vi "FF_compute2_Moiz.vi"(1 "GaitCylce(%)":dbl, 4 "Boolean":bool, 6 "FrameNum":dbl, 8 "xyz_o":dbl[][](array[numeric]), 10 "CenPt":dbl[](array[numeric]), 11 "Array":T1[](array[typedef])) -> (0 "Closest Pt":dbl[](array[numeric]), 2 "DesiredFM_FF":dbl[](array[numeric]), 3 "ForceAll":dbl[][](array[numeric]), 5 "curr Point":dbl[](array[numeric]), 9 "TraFF":dbl[](array[numeric]))   [LabVIEW 2013]
uses:
  typeDef/AnkleTraj.ctl
  <vilib>/Analysis/baseanly.llb/Real Dot Product.vi
  <vilib>/Analysis/_algsub.llb/Real Vector Norm.vi
  <vilib>/Analysis/BLAS.llb/idamin - Min Element Index (DBL).vi
  <vilib>/Analysis/NI_AALBase.lvlib
  <vilib>/Analysis/NI_AALPro.lvlib
  <vilib>/Analysis/NI_AALBLAS.lvlib
panel:
  out "Out of first loop":T1[](array[typedef])
  in  "FF Constant":T2
  in  "HalfWindow FF 2":i32=60
  out "x < y?":bool
  out "Array 2":i32[](array[numeric])
  out "P1FF":dbl[](array[numeric])
  out "P1 full size":i32[](array[numeric])
  out "P2 full":dbl[][](array[numeric])
  out "P1 full":dbl[][](array[numeric])
  out "CheckPlus":dbl[][](array[numeric])
  in  "AnkleTraj":T1
  out "HalfWindow FF":i32
  out "P'":dbl[](array[numeric])
  out "Array 4":dbl[](array[numeric])
  out "OrderOfClosePt":i32
  in  "DesiredM_FF":dbl[](array[numeric])=[5.0, 5.0, 5.0, 4.0, 4.0, 4.0]
  in  "Enum":enum16{"Linear", "Bell"}(ring)=enum."Bell"
  out "ForceComp":dbl[](array[numeric])
  out "n_dir":dbl[](array[numeric])
  out "d_min":dbl
  out "ForceXYZ":dbl[](array[numeric])
  out "TangentVectorAtClosestPt":dbl[](array[numeric])
  out "NormalVectorToClosestPt":dbl[](array[numeric])
  out "DistanceToClosestPt":dbl
  out "IndexOfClosePt":i32
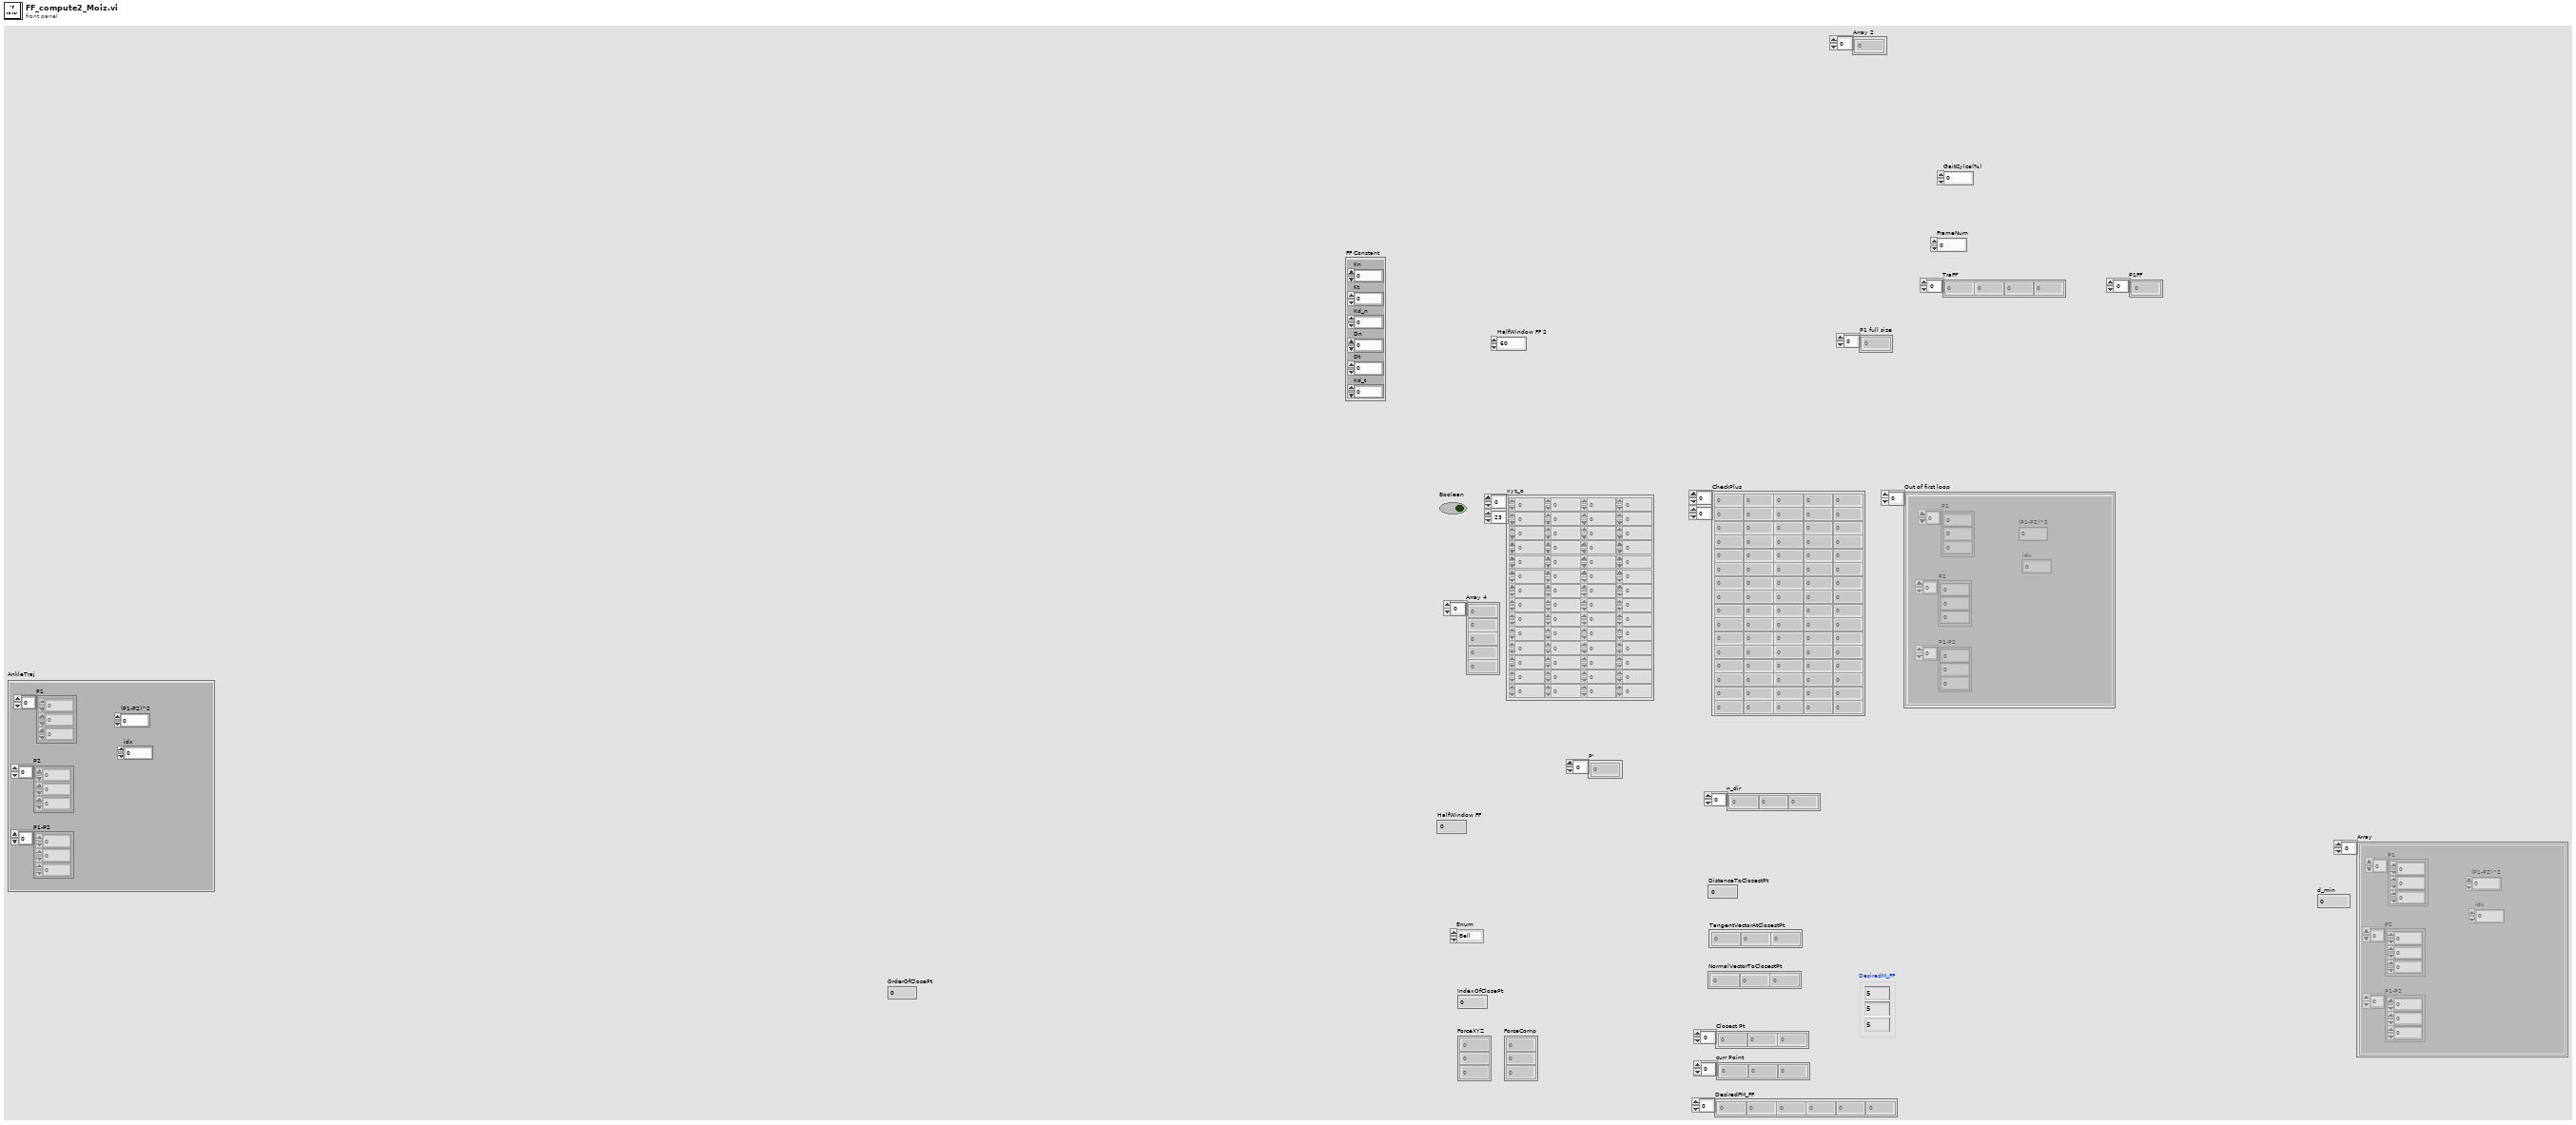
[diagram p1: front panel]
types:
  T1 = typedef "AnkleTraj.ctl" = cluster{"P1":dbl[], "P2":dbl[], "P1-P2":dbl[], "(P1-P2)^2":dbl, "idx":i32}
  T2 = cluster{"Kn":dbl, "Kt":dbl, "Kd_n":dbl, "Dn":dbl, "Dt":dbl, "Kd_t":dbl}
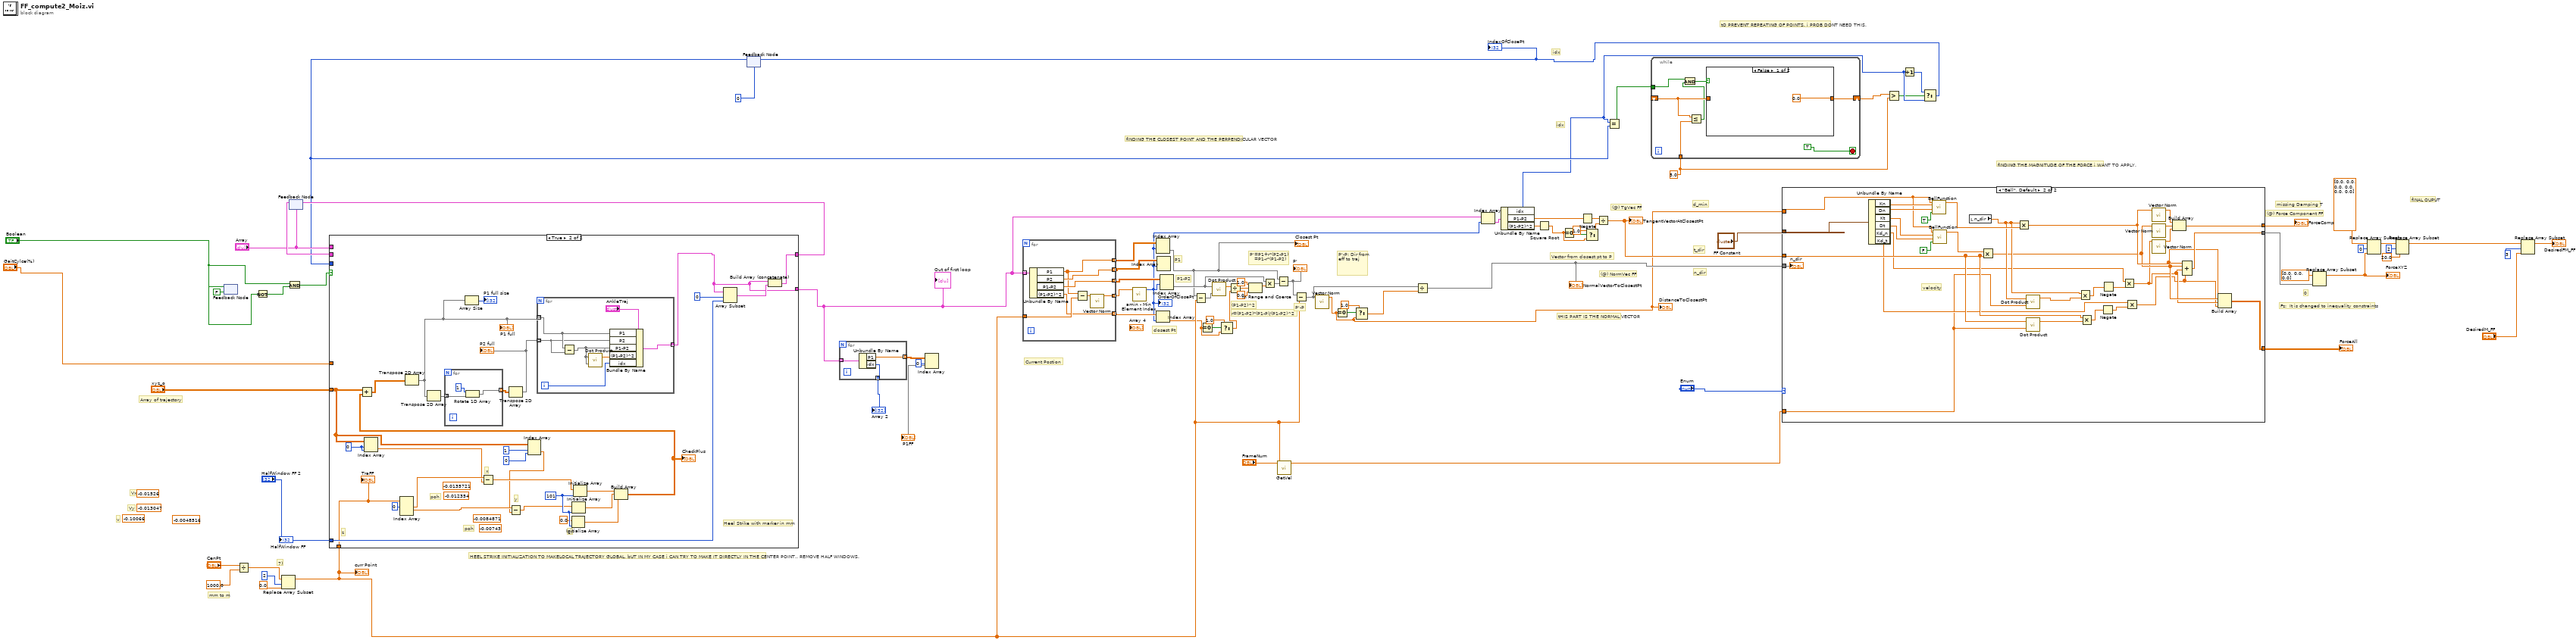
[diagram p0: block diagram]
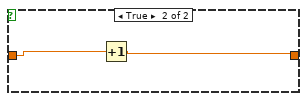
[diagram p2: hidden frame]
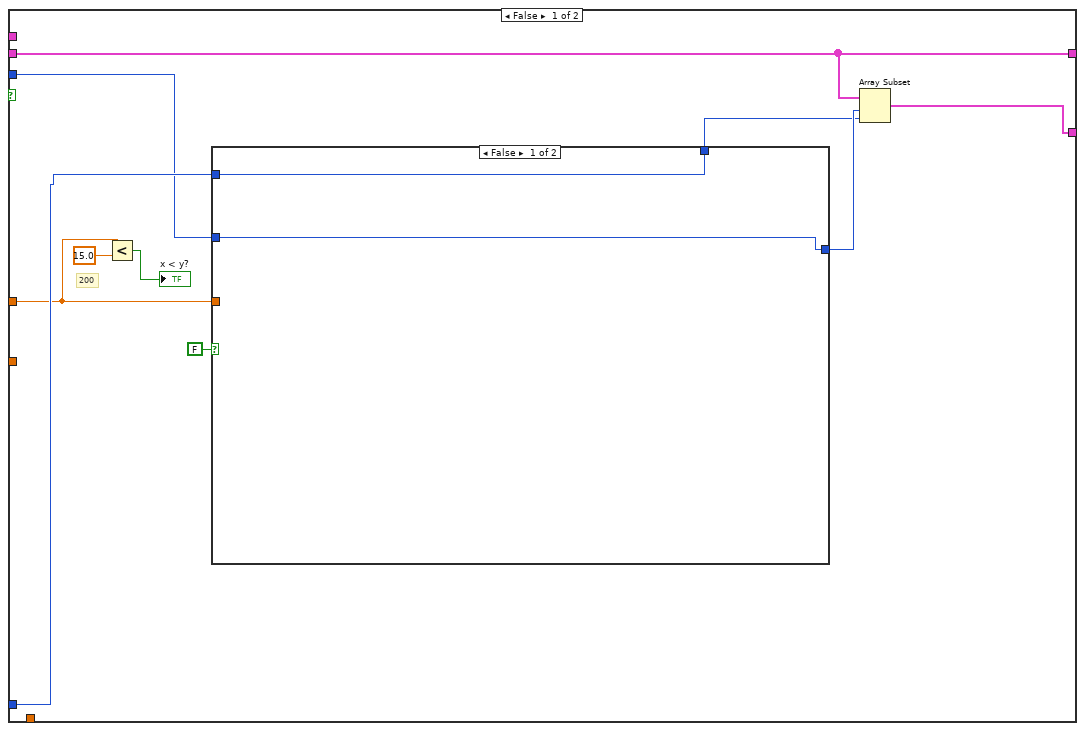
[diagram p3: hidden frame]
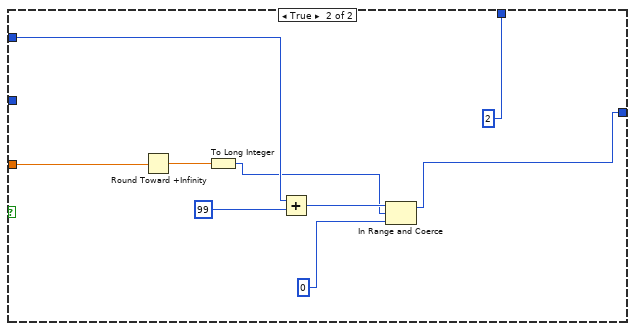
[diagram p4: hidden frame]
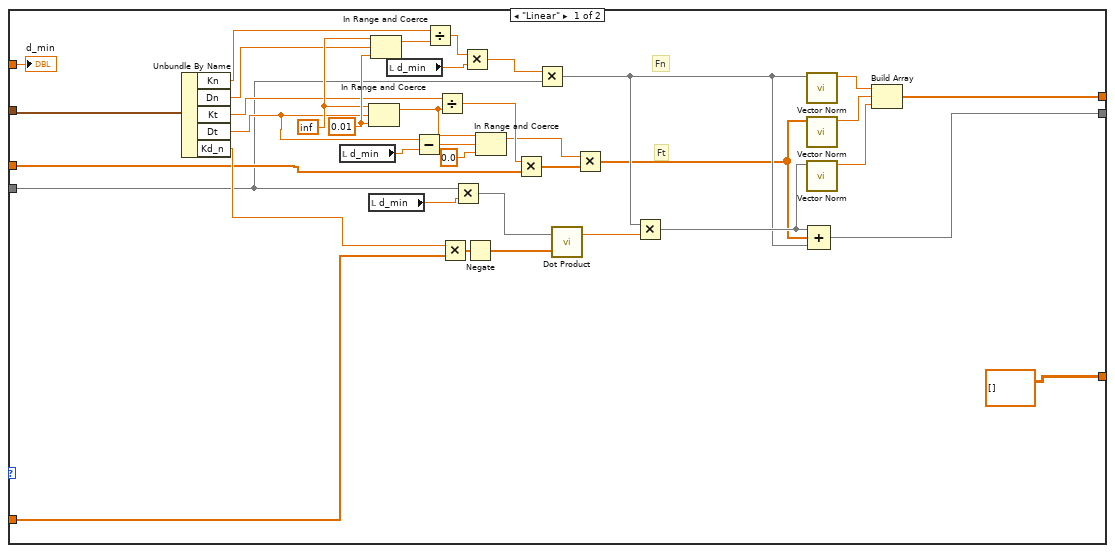
[diagram p5: hidden frame]
diagram:
  (unwired) -0.0048516 ("y")
  (unwired) -0.10066
  (unwired) -0.013047
  (unwired) -0.01526
  w16 = 5.0 ("y")
  # "fINAL OUPUT"
  # "tHIS PART IS THE NORMAL VECTOR"
  # "fINDING THE MAGNITUDE OF THE FORCE i WANT TO APPLY."
  # "tO PREVENT REPEATING OF POINTS. i PROB DONT NEED THIS."
  # "fINDING THE CLOSEST POINT AND THE PERPENDICULAR VECTOR"
  # "HEEL STRIKE INITIALIZATION TO MAKELOCAL TRAJECTORY GLOBAL. bUT IN MY CASE i CAN TRY TO MAKE IT DIRECTLY IN THE CENTER POINT.. REMOVE HALF WINDOWS."
  # "v"
  # "Vy"
  # "Vx"
  # "mm to m"
  # "idx"
  # "idx"
  # "missing Damping T"
  # "0"
  # "Fz:  It is changed to inequality constraints"
  # "(@) Force Component FF"
  # "(@) NormVec FF"
  # "(@) TgVec FF"
  # "Array of trajectory"
  # "7)"
  # "(P1-P2)^2"
  # "closest Pt"
  # "P1-P2"
  # "P1"
  # "P'-P"
  # "P'-P: Dir from eff to traj"
  # "r=(P1-P2)*(P1-P)/(P1-P2)^2"
  # "P'=P1+r*(P2-P1)\n   =P1-r*(P1-P2)"
  # "Current Postion"
  # "t_dir"
  # "n_dir"
  # "d_min"
  # "Vector from closest pt to P"
  n1 = feedback #1(FALSE ("Boolean")) -> (w42:bool)
  n2 = feedback-in #1("Boolean") -> ()
  n3 = Divide(x="CenPt", y=1000.0) -> (x/y=w39:dbl[])
  n4 = Not(x=w42) -> (.not. x?=w45:bool)
  n5 = Replace Array Subset(array=w39, new element=0.0 ("new element/subarray"), index=2) -> (w29:dbl[])
  "curr Point" <- w29
  n6 = And(x="Boolean", y=w45) -> (x .and. y?=w43:bool)
  n7 = feedback #2("Array") -> (w83:T1[])
  n8 = feedback #3(0) -> (w23:i32)
  n9 = case shown="True" w43 {
    tunnel: w23 -> [w88 _]
    tunnel: w83 -> [w94 _]
    tunnel: [w93 w128] -> w67
    tunnel: [w94 w133] -> w68
    tunnel: "Array" -> [_ _]
    tunnel: "HalfWindow FF 2" -> [w90 w132]
    tunnel: "xyz_o" -> [_ w109]
    tunnel: w29 -> [_ w112]
    tunnel: "GaitCylce(%)" -> [w87 _]
    frame False {
      # "200"
      n10 = Less?(x=w87, y=15.0) -> (x < y?=→"x < y?":bool)
      n11 = case shown="False" FALSE {
        tunnel: [w96 w104] -> w92
        tunnel: w88 -> [w96 _]
        tunnel: [w95 2] -> w91
        tunnel: w90 -> [w95 w103]
        tunnel: w87 -> [_ w99]
        frame False {
        }
        frame True {
          n12 = Round Toward +Infinity(x=w99) -> (ceil(x): smallest int >= x=w98:dbl)
          n13 = To Long Integer(number=w98) -> (32bit integer=w97:i32)
          n14 = Add(x=w103, y=99) -> (x+y=w102:i32)
          n15 = In Range and Coerce(upper limit=w102, x=w97, lower limit=0) -> (coerced(x)=w104:i32)  [unwired: 1 out]
        }
      }
      n16 = Array Subset(array=w94, index=w92, length=w91) -> (w93:T1[])
    }
    frame True {
      w111 = 0 ("index (row)")
      (unwired) -0.00743 ("x")
      (unwired) -0.012354 ("x")
      (unwired) -0.0084871 ("x")
      (unwired) -0.0135721 ("x")
      w126 = 101 ("dimension size")
      # "poh"
      # "poh"
      # "z"
      # "y"
      # "x"
      # "6)"
      # "Heel Strike with marker in mm"
      n17 = Index Array(array=w109, index (row)=w111, index (col)=w111) -> (element=w110:dbl)
      n18 = Index Array(array=w112, index #1=0 ("index")) -> (element #1=w118:dbl, element #2=w120:dbl)  [unwired: 2 in, 1 out]
      n19 = Subtract(x=w118, y=w110) -> (x-y=w117:dbl)
      n20 = Index Array(array=w109, index (row)=1 ("disabled index (col)"), index (col)=0 ("index (row)")) -> (element=w108:dbl)
      n21 = Subtract(x=w120, y=w108) -> (x-y=w119:dbl)
      n22 = Initialize Array(0.0 ("element"), w126) -> (w124:dbl[])
      n23 = Initialize Array(w119, w126) -> (w125:dbl[])
      n24 = Initialize Array(w117, w126) -> (w116:dbl[])
      n25 = Build Array(w116, w125, w124) -> (w123:dbl[][])
      "CheckPlus" <- w123
      n26 = Add(x=w109, y=w123) -> (x+y=w122:dbl[][])
      n27 = Transpose 2D Array(2D array=w122) -> (transposed array=w115:dbl[][])
      "P1 full" <- w115
      n28 = Transpose 2D Array(2D array=w115) -> (transposed array=w130:dbl[][])
      n29 = for {
        tunnel: w130 -> [w144] mode=indexing
        tunnel: [w143] -> w129 mode=indexing
        n30 = Rotate 1D Array(1:w144, 2:1 ("n")) -> (0:w143:dbl[])
      }
      n31 = Array Size(array=w115) -> (size(s)=→"P1 full size":i32[])
      n32 = Transpose 2D Array(2D array=w129) -> (transposed array=w113:dbl[][])
      "P2 full" <- w113
      n33 = for {
        tunnel: w115 -> [w140] mode=indexing
        tunnel: w113 -> [w139] mode=indexing
        tunnel: [w136] -> w128 mode=indexing
        i -> [w135]
        n34 = Subtract(x=w140, y=w139) -> (x-y=w137:dbl[])
        n35 = call-poly <vilib>:"Dot Product.vi"("Y Vector"=w137, "X Vector"=w137) -> ("X * Y"=w138:dbl)  [unwired: 1 out]
        n36 = Bundle By Name(cluster="AnkleTraj", "P1"=w140, "P2"=w139, "P1-P2"=w137, "(P1-P2)^2"=w138, "idx"=w135) -> (w136:T1)
      }
      n37 = Array Subset(array=w128, index=0, length=w132) -> (w134:T1[])
      n38 = Build Array (concatenate)(w128, w134) -> (w133:T1[])
      "TraFF" <- w112
    }
  }
  "Out of first loop" <- w67
  n39 = feedback-in #2(w68) -> ()
  n40 = for {
    tunnel: w67 -> [w147] mode=indexing
    tunnel: [w146] -> w36 mode=indexing
    tunnel: [w145] -> w25 mode=indexing
    n41 = Unbundle By Name(w147) -> ("P1"=w146:dbl[], "idx"=w145:i32)
  }
  "Array 2" <- w25
  n42 = Index Array(array=w36, index (row)=0) -> (element=→"P1FF":dbl[])  [unwired: 1 in]
  n43 = for {
    tunnel: w67 -> [w155] mode=indexing
    tunnel: w29 -> [w152]
    tunnel: [w151] -> w52 mode=indexing
    tunnel: [w154] -> w51 mode=indexing
    tunnel: [w153] -> w50 mode=indexing
    tunnel: [w150] -> w49 mode=indexing
    tunnel: [w148] -> w47 mode=indexing
    n44 = Unbundle By Name(w155) -> ("P1"=w151:dbl[], "P2"=w154:dbl[], "P1-P2"=w153:dbl[], "(P1-P2)^2"=w150:dbl)
    n45 = Subtract(x=w151, y=w152) -> (x-y=w149:dbl[])
    n46 = call-poly <vilib>:"Vector Norm.vi"("Input Vector"=w149) -> ("norm"=w148:dbl)  [unwired: 9 in, 1 out]
  }
  n47 = call-poly <vilib>:"amin - Min Element Index.vi"("x"=w47) -> ("idamin"=w26:i32)  [unwired: 9 in, 1 out]
  "OrderOfClosePt" <- w26
  n48 = Index Array(array=w52, index (row)=w26) -> (element=w24:dbl[])  [unwired: 1 in]
  "Closest Pt" <- w24
  n49 = Index Array(array=w49, index=w26) -> (element=w5:dbl)
  n50 = Index Array(array=w51, index (row)=w26) -> ()  [unwired: 1 in, 1 out]
  n51 = Index Array(array=w50, index (row)=w26) -> (element=w55:dbl[])  [unwired: 1 in]
  n52 = Subtract(x=w24, y=w29) -> (x-y=w62:dbl[])
  n53 = Equal To 0?(x=w5) -> (x = 0?=w7:bool)
  n54 = call-poly <vilib>:"Dot Product.vi"("Y Vector"=w62, "X Vector"=w55) -> ("X * Y"=w61:dbl)  [unwired: 1 out]
  n55 = Select(t=1.0, s=w7, f=w5) -> (s? t:f=w4:dbl)
  n56 = Divide(x=w61, y=w4) -> (x/y=w60:dbl)
  n57 = In Range and Coerce(upper limit=1.0, x=w60, lower limit=0.0) -> (coerced(x)=w57:dbl)  [unwired: 1 out]
  n58 = Multiply(x=w55, y=w57) -> (x*y=w56:dbl[])
  n59 = Subtract(x=w24, y=w56) -> (x-y=w53:dbl[])
  "P'" <- w53
  n60 = call "GetVel.vi"("Position"=w29, "FrameNum"="FrameNum") -> ("Velocity"=w30:dbl[])  [unwired: 9 in]
  n61 = Subtract(x=w53, y=w29) -> (x-y=w54:dbl[])
  n62 = call-poly <vilib>:"Vector Norm.vi"("Input Vector"=w54) -> ("norm"=w3:dbl)  [unwired: 9 in, 1 out]
  "DistanceToClosestPt" <- w3
  n63 = Equal To 0?(x=w3) -> (x = 0?=w14:bool)
  n64 = Select(t=1.0, s=w14, f=w3) -> (s? t:f=w12:dbl)
  n65 = Divide(x=w54, y=w12) -> (x/y=w48:dbl[])
  "NormalVectorToClosestPt" <- w48
  n66 = Index Array(array=w67, index=w26) -> (element=w76:T1)
  n67 = Unbundle By Name(w76) -> ("idx"=w22:i32, "P1-P2"=w78:dbl[], "(P1-P2)^2"=w79:dbl)
  n68 = Square Root(x=w79) -> (sqrt(x)=w9:dbl)
  n69 = Equal To 0?(x=w9) -> (x = 0?=w11:bool)
  n70 = Negate(x=w78) -> (-x=w77:dbl[])
  n71 = Select(t=1.0, s=w11, f=w9) -> (s? t:f=w8:dbl)
  n72 = Divide(x=w77, y=w8) -> (x/y=w63:dbl[])
  "TangentVectorAtClosestPt" <- w63
  n73 = Equal?(x=w22, y=w23) -> (x = y?=w20:bool)
  n74 = while {
    tunnel: w20 -> [w159]
    shift-right: [w162] -> w18
    shift-left: _ -> [w160]
    tunnel: w16 -> [w156]
    stop <- TRUE stop-if-true
    n75 = Less Or Equal?(x=w160, y=w156) -> (x <= y?=w158:bool)
    n76 = And(x=w159, y=w158) -> (x .and. y?=w157:bool)
    n77 = case shown="False" w157 {
      tunnel: [0.0 w164] -> w162
      tunnel: w160 -> [_ w165]
      frame False {
      }
      frame True {
        n78 = Increment(x=w165) -> (x+1=w164:dbl)
      }
    }
  }
  n79 = case shown="\"Bell\", Default" "Enum" {
    tunnel: [w202 w230] -> w64
    tunnel: [w181 w234] -> w80
    tunnel: w30 -> [w201 w208]
    tunnel: "FF Constant" -> [w180 w229]
    tunnel: w63 -> [w174 w216]
    tunnel: w3 -> [w172 w220]
    tunnel: w48 -> [w173 w221]
    tunnel: [dbl[][] [] w203] -> w28
    frame "Linear" {
      w186 = inf
      w187 = 0.01 ("upper limit")
      # "Ft"
      # "Fn"
      n80 = Unbundle By Name(w180) -> ("Kn"=w179:dbl, "Dn"=w178:dbl, "Kt"=w177:dbl, "Dt"=w176:dbl, "Kd_n"=w175:dbl)
      n81 = local read "d_min"() -> (w170:dbl)
      n82 = In Range and Coerce(upper limit=w186, x=w176, lower limit=w187) -> (coerced(x)=w188:dbl)  [unwired: 1 out]
      n83 = local read "d_min"() -> (w169:dbl)
      n84 = In Range and Coerce(upper limit=w186, x=w178, lower limit=w187) -> (coerced(x)=w189:dbl)  [unwired: 1 out]
      n85 = local read "d_min"() -> (w171:dbl)
      n86 = Subtract(x=w176, y=w170) -> (x-y=w192:dbl)
      n87 = Divide(x=w179, y=w189) -> (x/y=w185:dbl)
      n88 = Divide(x=w177, y=w188) -> (x/y=w190:dbl)
      n89 = Multiply ("Multiply.vi")(x=w175, y=w201) -> (x*y=w197:dbl[])
      n90 = Multiply(x=w173, y=w169) -> (x*y=w196:dbl[])
      n91 = Multiply(x=w185, y=w171) -> (x*y=w184:dbl)
      n92 = Negate(x=w197) -> (-x=w195:dbl[])
      n93 = In Range and Coerce(upper limit=w188, x=w192, lower limit=0.0) -> (coerced(x)=w167:dbl)  [unwired: 1 out]
      n94 = Multiply(x=w190, y=w174) -> (x*y=w193:dbl[])
      n95 = Multiply(x=w184, y=w173) -> (x*y=w182:dbl[])
      n96 = call-poly <vilib>:"Dot Product.vi"("Y Vector"=w195, "X Vector"=w196) -> ("X * Y"=w194:dbl)  [unwired: 1 out]
      n97 = Multiply(x=w167, y=w193) -> (x*y=w168:dbl[])
      n98 = Multiply(x=w182, y=w194) -> (x*y=w183:dbl[])
      n99 = call-poly <vilib>:"Vector Norm.vi"("Input Vector"=w182) -> ("norm"=w198:dbl)  [unwired: 9 in, 1 out]
      n100 = call-poly <vilib>:"Vector Norm.vi"("Input Vector"=w168) -> ("norm"=w199:dbl)  [unwired: 9 in, 1 out]
      n101 = call-poly <vilib>:"Vector Norm.vi"("Input Vector"=w183) -> ("norm"=w200:dbl)  [unwired: 9 in, 1 out]
      n102 = Compound Arithmetic op=ADD(w183, w168, w182) -> (w181:dbl[])
      n103 = Build Array(w198, w199, w200) -> (w202:dbl[])
      "d_min" <- w172
    }
    frame "Bell", Default {
      # "velocity"
      n104 = Unbundle By Name(w229) -> ("Kn"=w223:dbl, "Dn"=w224:dbl, "Kt"=w225:dbl, "Dt"=w226:dbl, "Kd_n"=w212:dbl, "Kd_t"=w209:dbl)
      n105 = call "BellFunction.vi"("Invert"=TRUE, "(r)adius"=w224, "(A)mplitude"=w223, "x"=w220) -> ("y"=w219:dbl)  [unwired: 2 in]
      n106 = call "BellFunction.vi"("Invert"=FALSE, "(r)adius"=w226, "(A)mplitude"=w225, "x"=w220) -> ("y"=w222:dbl)  [unwired: 2 in]
      n107 = local read "n_dir"() -> (w217:dbl[])
      n108 = Multiply(x=w222, y=w216) -> (x*y=w206:dbl[])
      n109 = Multiply(x=w217, y=w219) -> (x*y=w207:dbl[])
      n110 = call-poly <vilib>:"Dot Product.vi"("Y Vector"=w208, "X Vector"=w217) -> ("X * Y"=w218:dbl)  [unwired: 1 out]
      n111 = call-poly <vilib>:"Dot Product.vi"("Y Vector"=w208, "X Vector"=w216) -> ("X * Y"=w215:dbl)  [unwired: 1 out]
      n112 = Multiply(x=w217, y=w218) -> (x*y=w214:dbl[])
      n113 = Multiply(x=w216, y=w215) -> (x*y=w213:dbl[])
      n114 = Negate(x=w213) -> (-x=w210:dbl[])
      n115 = Negate(x=w214) -> (-x=w211:dbl[])
      n116 = Multiply(x=w212, y=w211) -> (x*y=w205:dbl[])
      n117 = Multiply(x=w209, y=w210) -> (x*y=w204:dbl[])
      n118 = call-poly <vilib>:"Vector Norm.vi"("Input Vector"=w207) -> ("norm"=w233:dbl)  [unwired: 9 in, 1 out]
      n119 = call-poly <vilib>:"Vector Norm.vi"("Input Vector"=w206) -> ("norm"=w232:dbl)  [unwired: 9 in, 1 out]
      n120 = call-poly <vilib>:"Vector Norm.vi"("Input Vector"=w205) -> ("norm"=w231:dbl)  [unwired: 9 in, 1 out]
      n121 = Build Array(w233, w232, w231) -> (w230:dbl[])
      n122 = Compound Arithmetic op=ADD(w207, w206, w205, w204) -> (w234:dbl[])
      n123 = Build Array(w207, w206, w205, w204) -> (w203:dbl[][])
      "n_dir" <- w221
    }
  }
  "ForceComp" <- w64
  "ForceAll" <- w28
  n124 = Greater?(x=w18, y=w16) -> (0:w17:bool)
  n125 = Increment(x=w22) -> (x+1=w19:i32)
  n126 = Select(t=w19, s=w17, f=w22) -> (s? t:f=w21:i32)
  "IndexOfClosePt" <- w21
  n127 = feedback-in #3(w21) -> ()
  n128 = Replace Array Subset(array=dbl[] [0.0, 0.0, 0.0], new element=w80) -> (w65:dbl[])  [unwired: 1 in]
  "ForceXYZ" <- w65
  n129 = Replace Array Subset(array=dbl[] [0.0, 0.0, 0.0, 0.0, 0.0, 0.0] ("element"), new element=w65, index=0) -> (w33:dbl[])
  n130 = Replace Array Subset(array=w33, new element=20.0 ("new element/subarray"), index=2) -> (w32:dbl[])
  n131 = Replace Array Subset(array=w32, new element="DesiredM_FF", index=3) -> (→"DesiredFM_FF":dbl[])
  "HalfWindow FF" <- "HalfWindow FF 2"
